vi "Main.vi"(5 "Deliminated Char":string=".", 6 "Folder names":string[](array[string])=["StaARx#[PLC]StaATesterRxSignals", "StaATx#[PLC]StaATesterTxSignals"], 7 "FGVname":string="OPC Ref", 8 "error in":errorcluster, 9 "Sequence Context In":refnum<k7>, 10 "Event Sources":T1, 11 "OPC UA In":refnum<class "OPC UA.lvclass">) -> (0 "error out":errorcluster, 2 "Station":string="asdfasdf", 3 "OPC UA Out":refnum<class "OPC UA.lvclass">)   [LabVIEW 2021, in "OPC UA.lvlib" / "OPC UA.lvclass"]
uses:
  OPC UA.lvclass
  <vilib>/OPCUA/controls/OPC UA Client Refnum.ctl
  OPC UA.lvclass/OPC UA.ctl
  <vilib>/OPCUA/NI OPC UA Client.lvlib
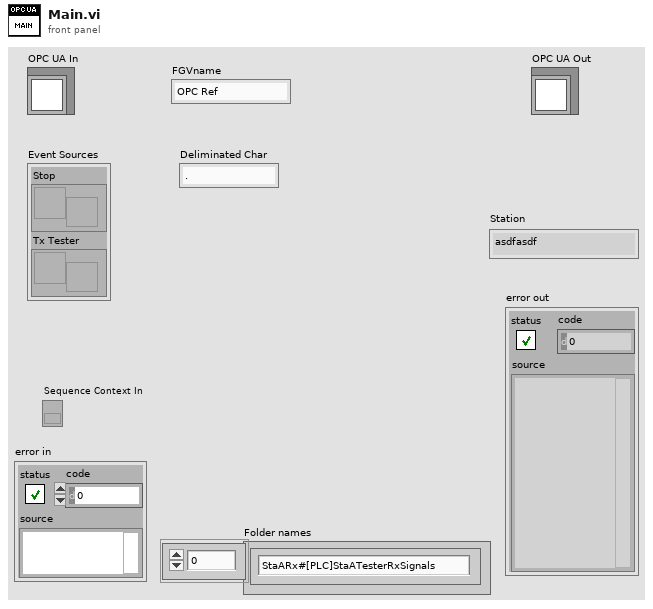
[diagram p1: front panel]
types:
  T1 = cluster{"Stop":refnum<user-event>, "Tx Tester":refnum<user-event>}
  T2 = typedef "OPC UA Client Refnum.ctl" = refnum<k21>
  T3 = typedef "Subscription ID.ctl" = u32
  T4 = typedef "TestStand - Status Monitor.ctl" = cluster{"Sequence Context":refnum<k7>, "Execution":refnum<k7>, "Termination Monitor":refnum<k7>}
  T5 = cluster{"Event Registration Refnum":refnum<event-registration>, "Event Registration Refnum":refnum<event-registration>}
  T6 = typedef "Subscription Data Change.ctl" = cluster{"node ID":T7, " value":variant, "timestamp":timestamp, "data type":T8, "status code":T9}
  T7 = typedef "NodeId.ctl" = string
  T8 = typedef "Data Type.ctl" = u16
  T9 = typedef "OPC UA StatusCode.ctl" = u32
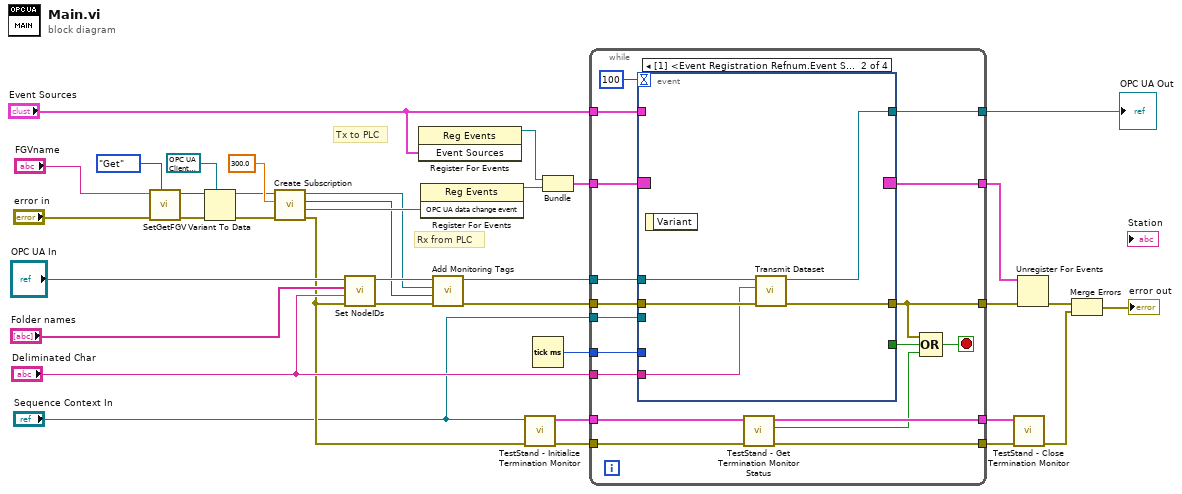
[diagram p0: block diagram]
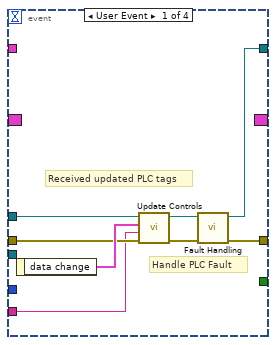
[diagram p2: hidden frame]
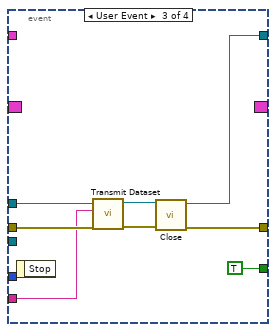
[diagram p3: hidden frame]
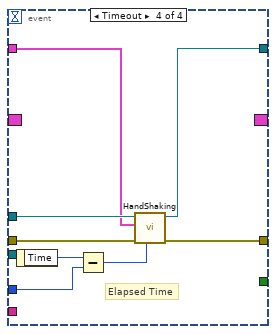
[diagram p4: hidden frame]
diagram:
  # "Tx to PLC"
  # "Rx from PLC"
  n1 = call "SetGetFGV.vi"("Method (Get)"=enum16{"Get", "Set"}."Get", "error in"="error in", "Name"="FGVname") -> ("error out"=w12:errorcluster, "Data out"=w9:variant)  [unwired: 7 in]
  n2 = Variant To Data(error in=w12, type=T2 refnum ("OPC UA client refnum out"), Variant=w9) -> (data=w7:T2, error out=w6:errorcluster)
  n3 = call <vilib>:"Create Subscription.vi"("error in (no error)"=w6, "publishing interval (1000 ms)"=300.0, "OPC UA client refnum in"=w7) -> ("error out"=w2:errorcluster, "OPC UA data change event"=w18:refnum<user-event>, "subscription ID out"=w17:T3, "OPC UA client refnum out"=w16:T2)  [unwired: 4 in, 1 out]
  n4 = call "Set NodeIDs.vi"("error in (no error)"=w2, "Deliminated Char"="Deliminated Char", "PLC Folder Names"="Folder names", "OPC UA in"="OPC UA In") -> ("error out"=w35:errorcluster, "OPC UA out"=w34:refnum<class "OPC UA.lvclass">)  [unwired: 6 in]
  n5 = register-events("Event Sources") -> (reference out=w25:refnum<event-registration>)  [unwired: 2 in, 1 out]
  n6 = register-events(w18) -> (reference out=w26:refnum<event-registration>)  [unwired: 2 in, 1 out]
  n7 = call "Add Monitoring Tags.vi"("error in (no error)"=w35, "subscription ID"=w17, "OPC UA client refnum"=w16, "OPC UA in"=w34) -> ("error out"=w15:errorcluster, "OPC UAout"=w20:refnum<class "OPC UA.lvclass">)  [unwired: 6 in]
  n8 = call <vilib>:"TestStand - Initialize Termination Monitor.vi"("error in (no error)"=w2, "Sequence Context In"="Sequence Context In") -> ("error out"=w33:errorcluster, "Status Monitor Out"=w32:T4)  [unwired: 8 in]
  n9 = Tick Count (ms)() -> (millisecond timer value=w24:u32)
  n10 = Bundle("Event Registration Refnum"=w25, "Event Registration Refnum"=w26) -> (w5:T5)  [unwired: 1 in]
  n11 = while {
    tunnel: w5 -> [w54]
    tunnel: w20 -> [w53]
    tunnel: w15 -> [w52]
    tunnel: [w40] -> w29
    tunnel: [w50] -> w28
    tunnel: w33 -> [w49]
    tunnel: w32 -> [w48]
    tunnel: [w46] -> w31
    tunnel: [w45] -> w30
    tunnel: "Event Sources" -> [w44]
    tunnel: [w43] -> w14
    tunnel: w24 -> [w42]
    tunnel: "Deliminated Char" -> [w38]
    tunnel: "Sequence Context In" -> [w37]
    stop <- w47 stop-if-true
    n12 = event shown="[1] <Event Registration Refnum.Event Sources.Tx Tester>: User Event" {
      selector: w54 -> [_ _ _ _]
      dyn-events: [_ _ _ _] -> w50
      timeout: 100 -> [_ _ _ _]
      tunnel: w53 -> [w62 w65 w73 w81]
      tunnel: w52 -> [w60 w66 w72 w80]
      tunnel: [w58 w67 w75 w83] -> w40
      tunnel: w44 -> [_ _ _ w76]
      tunnel: [w57 w64 w74 w82] -> w43
      tunnel: w42 -> [_ _ _ w78]
      tunnel: [_ _ TRUE ("Stop") _] -> w39
      tunnel: w38 -> [w55 w63 w68 _]
      tunnel: w37 -> [_ _ _ _]
      event User Event {
        # "Handle PLC Fault"
        # "Received updated PLC tags"
        n13 = event-data() -> ("data change"=w61:T6[])  [unwired: 1 in]
        n14 = call "Update Controls.vi"("error in (no error)"=w60, "Deliminated Char"=w55, "data change"=w61, "OPC UA in"=w62) -> ("error out"=w59:errorcluster, "OPC UA out"=w56:refnum<class "OPC UA.lvclass">)  [unwired: 6 in]
        n15 = call-dynamic "Fault Handling.vi"("error in (no error)"=w59, "OPC UA in"=w56) -> ("error out"=w58:errorcluster, "OPC UA out"=w57:refnum<class "OPC UA.lvclass">)  [unwired: 7 in, 1 out]
      }
      event User Event {
        n16 = event-data() -> ()  [unwired: 1 in, 1 out]
        n17 = call "Transmit Dataset.vi"("error in (no error)"=w66, "Deliminator Char"=w63, "OPC UA in"=w65) -> ("error out"=w67:errorcluster, "OPC UA out"=w64:refnum<class "OPC UA.lvclass">)  [unwired: 7 in]
      }
      event User Event {
        n18 = event-data() -> ()  [unwired: 1 in, 1 out]
        n19 = call "Transmit Dataset.vi"("error in (no error)"=w72, "Deliminator Char"=w68, "OPC UA in"=w73) -> ("error out"=w70:errorcluster, "OPC UA out"=w71:refnum<class "OPC UA.lvclass">)  [unwired: 7 in]
        n20 = call-dynamic "Close.vi"("error in"=w70, "OPC UA in"=w71) -> ("error out"=w75:errorcluster, "OPC UA out"=w74:refnum<class "OPC UA.lvclass">)  [unwired: 8 in]
      }
      event Timeout {
        # "Elapsed Time"
        n21 = event-data() -> ("Time"=w79:u32)  [unwired: 1 in]
        n22 = Subtract(x=w79, y=w78) -> (x-y=w77:u32)
        n23 = call-dynamic "HandShaking.vi"("Elapsed Time"=w77, "error in (no error)"=w80, "Event Sources"=w76, "OPC UA in"=w81) -> ("error out"=w83:errorcluster, "OPC UA out"=w82:refnum<class "OPC UA.lvclass">)  [unwired: 6 in]
      }
    }
    n24 = call <vilib>:"TestStand - Get Termination Monitor Status.vi"("error in (no error)"=w49, "Status Monitor In"=w48) -> ("error out"=w46:errorcluster, "Terminating or Aborting"=w41:bool, "Status Monitor Out"=w45:T4)  [unwired: 7 in]
    n25 = Compound Arithmetic op=OR(w40, w39, w41) -> (w47:bool)
  }
  "OPC UA Out" <- w14
  n26 = call <vilib>:"TestStand - Close Termination Monitor.vi"("error in (no error)"=w31, "Status Monitor In"=w30) -> ("error out"=w22:errorcluster)  [unwired: 9 in]
  n27 = Unregister For Events(event registration refnum=w28, error in=w29) -> (error out=w23:errorcluster)
  n28 = Merge Errors(w23, w22) -> (→"error out":errorcluster)
